vi "Dequeue Element.vi"(6 "timeout in ms (-1)":i32=-1, 8 "error in (no error)":errorcluster, 9 "index":i32, 11 "Queue Array":T1) -> (0 "error out":errorcluster, 2 "Queue Element":T2, 3 "Queue Out":refnum<queue>)   [LabVIEW 2017]
uses:
  Queue Element.ctl
  Queue References Array.ctl
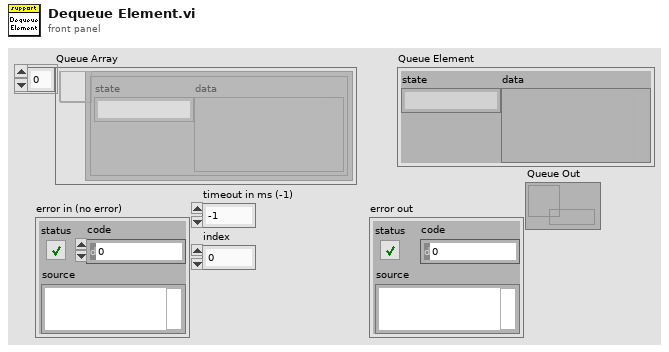
[diagram p1: front panel]
types:
  T1 = typedef "Queue References Array.ctl" = refnum<queue>[]
  T2 = typedef "Queue Element.ctl" = cluster{"state":string, "data":variant}
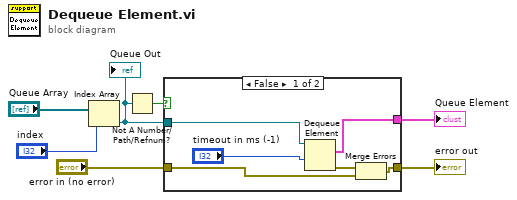
[diagram p0: block diagram]
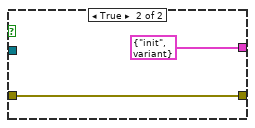
[diagram p2: hidden frame]
diagram:
  n1 = Index Array(array="Queue Array", index="index") -> (element=w4:refnum<queue>)
  "Queue Out" <- w4
  n2 = Not A Number/Path/Refnum?(number/path/refnum=w4) -> (NaN/Path/Refnum?=w2:bool)
  n3 = case shown="False" w2 {
    tunnel: [w13 T2 {"state"="init", "data"=variant} ("Queue Element")] -> w7
    tunnel: w4 -> [w12 _]
    tunnel: "error in (no error)" -> [w8 w15]
    tunnel: [w9 w15] -> w6
    frame False {
      n4 = Dequeue Element(queue=w12, timeout in ms (-1)="timeout in ms (-1)") -> (element=w13:T2, error out=w11:errorcluster)  [unwired: 1 in, 2 out]
      n5 = Merge Errors(w11, w8) -> (w9:errorcluster)
    }
    frame True {
    }
  }
  "Queue Element" <- w7
  "error out" <- w6
